vi "使用次数和硬盘序列号.vi"(0 "allowTimes":i32=10, 1 "使用期限":timestamp=timestamp(3494953806 s since 1904-01-01), 2 "serialNum":string, 3 "最小日期":timestamp=timestamp(3494953806 s since 1904-01-01)) -> (7 "curTimes":i32=1000, 8 "writen":bool, 9 "moreTimes":bool, 10 "moreUse":bool)   [LabVIEW 2010]
doc: "This example demonstrates how to write, read, and delete a sample key from the Windows registry. It will not affect the registry in any other way."
uses:
  <vilib>/registry/registry.llb/Registry RtKey.ctl
  <vilib>/registry/registry.llb/Read Registry Value Simple STR.vi
  <vilib>/registry/registry.llb/Write Registry Value Simple STR.vi
  kernel32.dll
  hdd/GetHW.dll
panel:
  out "CPU Manufacturers":string
  out "CPU Specification":string
  out "CPU SN":string
  out "错误输出 3":errorcluster caption="错误输出"
  out "最小日期":bool
  out "未超过使用期限":bool
  out "当前时间":timestamp
  out "Sample Key Deleted?":bool
  in  "清空注册表记录":bool
  out "same":bool
  out "error out":errorcluster caption="错误输出"
  out "硬盘序列号":string
  out "数值 3":i32=12
  out "数值":i32=12
  out "return type":string
  out "已经使用次数":string="My String"
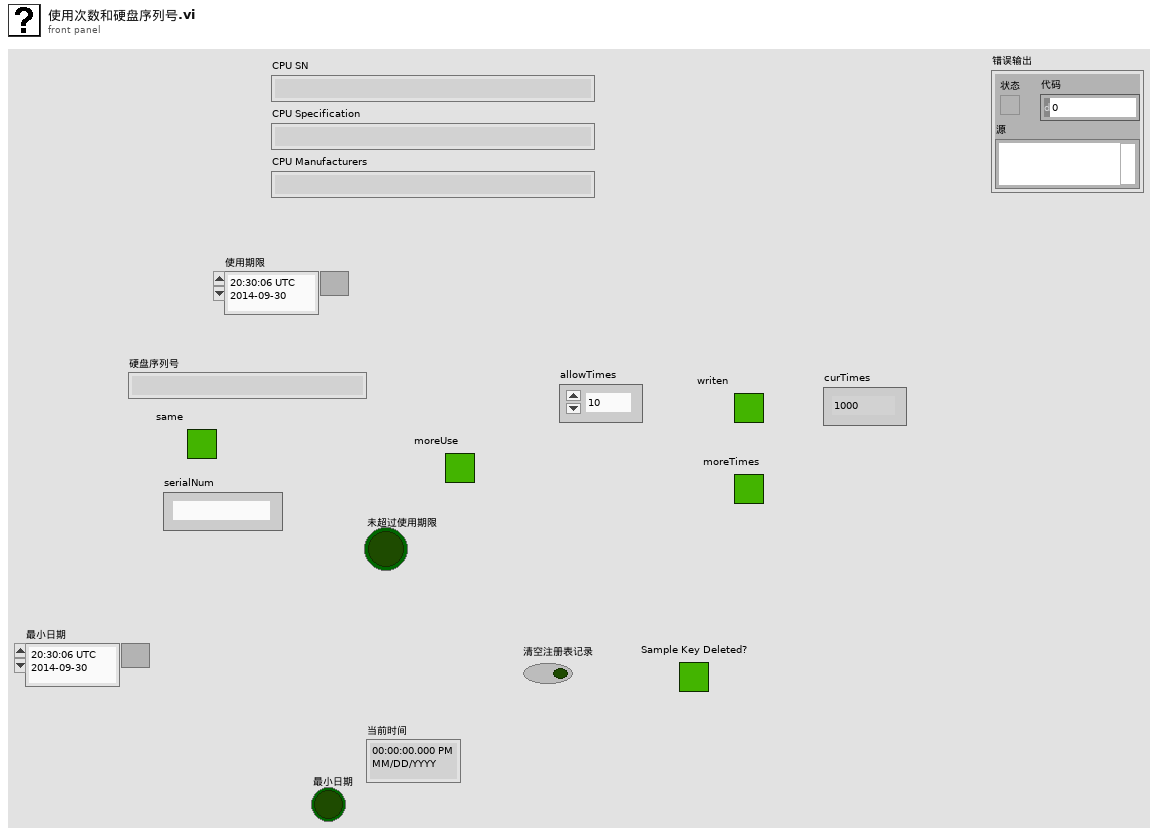
[diagram p1: front panel]
types:
  T1 = typedef "Registry RtKey.ctl" = enum32{"HKEY_CLASSES_ROOT", "HKEY_CURRENT_USER", "HKEY_LOCAL_MACHINE", "HKEY_USERS", "HKEY_PERFORMANCE_DATA", "HKEY_CURRENT_CONFIG", "HKEY_DYN_DATA"}
  T2 = typedef "Registry refnum.ctl" = refnum<k1>
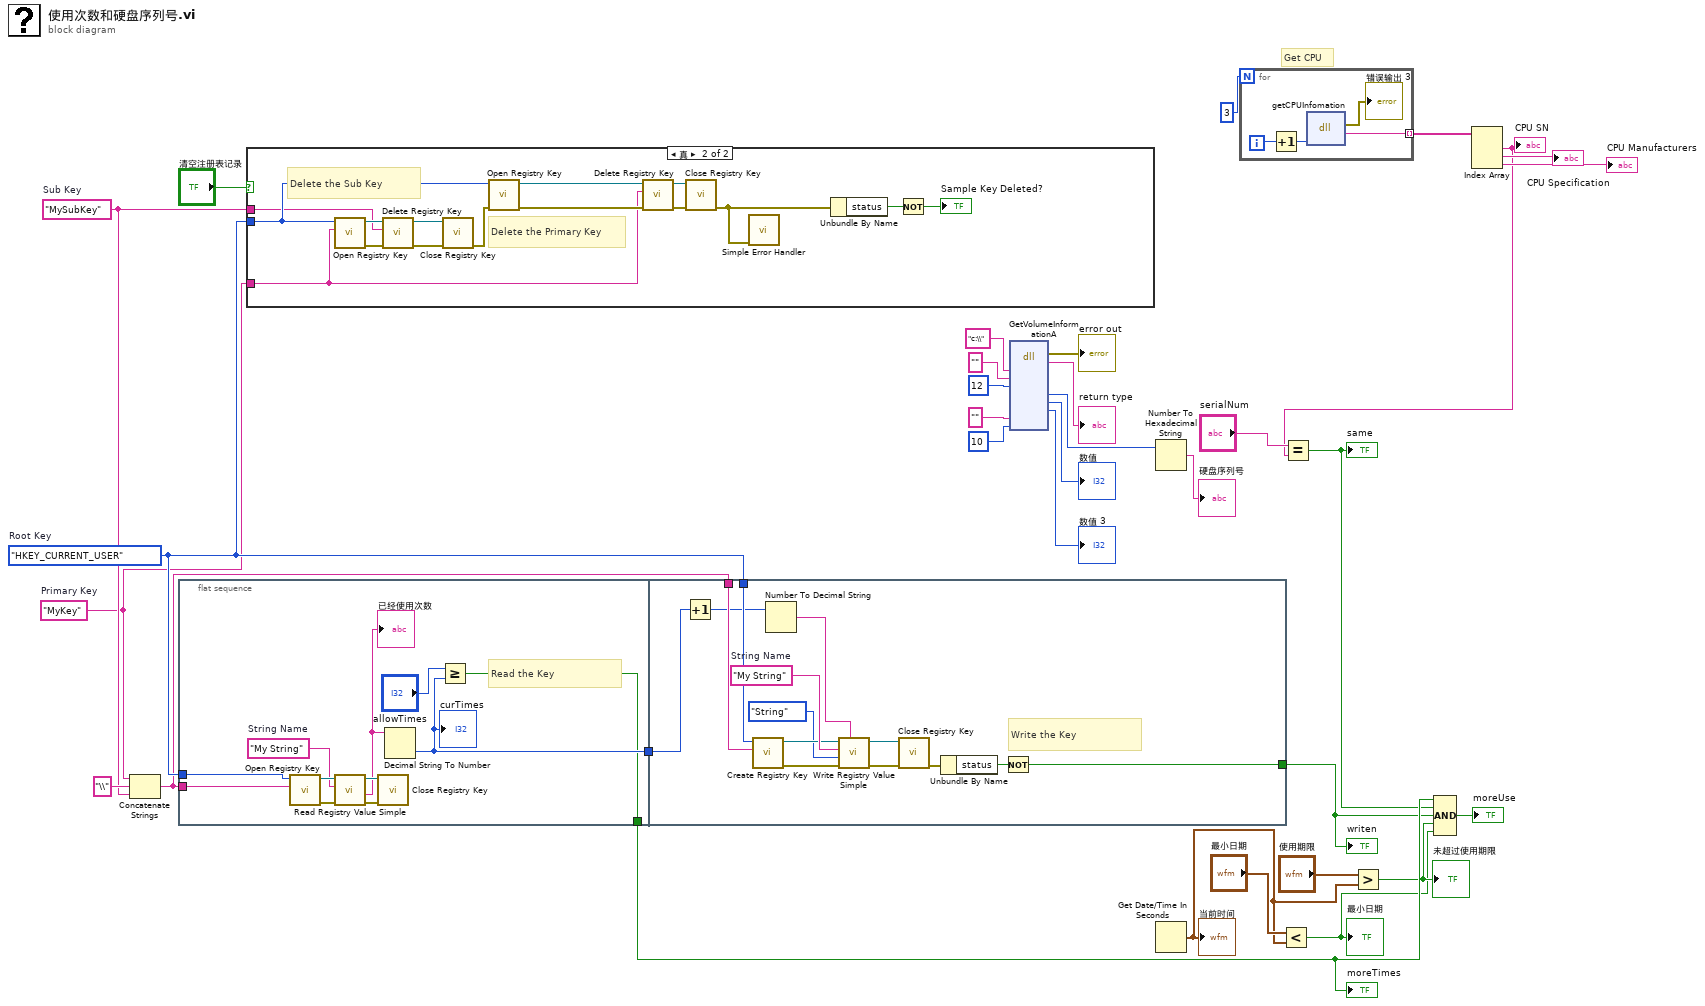
[diagram p0: block diagram]
diagram:
  w15 = "MySubKey"  # Sub Key
  w13 = "MyKey"  # Primary Key
  w17 = Registry_RtKey."HKEY_CURRENT_USER"  # Root Key
  # "Get CPU"
  n1 = Concatenate Strings(w13, "\\", w15) -> (w14:string)
  n2 = flat-sequence {
    tunnel: w17 -> [w39]
    tunnel: w14 -> [w38]
    tunnel: [w35] -> w33
    tunnel: [w34] -> w21
    tunnel: w33 -> [w58]
    tunnel: w14 -> [w50]
    tunnel: w17 -> [w49]
    tunnel: [w46] -> w18
    frame #0 {
      w40 = "My String"  # String Name
      # "Read the Key"
      n3 = call <vilib>:"Open Registry Key.vi"("subkey"=w38, "root key (HKEY_LOCAL_MACHINE)"=w39) -> ("error out"=w41:errorcluster, "refnum out"=w42:T2)  [unwired: 8 in]
      n4 = call-poly <vilib>:"Read Registry Value Simple.vi"("error in (no error)"=w41, "value"=w40, "refnum"=w42) -> ("error out"=w44:errorcluster, "String/Binary data"=w36:string, "refnum out"=w43:T2)  [unwired: 3 in, 1 out]
      "已经使用次数" <- w36
      n5 = call <vilib>:"Close Registry Key.vi"("error in (no error)"=w44, "refnum"=w43) -> ()  [unwired: 5 in, 1 out]
      n6 = Decimal String To Number(string=w36) -> (number=w35:i32)  [unwired: 2 in, 1 out]
      "curTimes" <- w35
      n7 = Greater Or Equal?(x="allowTimes", y=w35) -> (x >= y?=w34:bool)
    }
    frame #1 {
      w57 = "My String"  # String Name
      # "Write the Key"
      n8 = Increment(x=w58) -> (x+1=w48:i32)
      n9 = call <vilib>:"Create Registry Key.vi"("subkey"=w50, "root key (HKEY_LOCAL_MACHINE)"=w49) -> ("error out"=w53:errorcluster, "refnum out"=w55:T2)  [unwired: 7 in, 1 out]
      n10 = Number To Decimal String(number=w48) -> (decimal integer string=w47:string)  [unwired: 1 in]
      n11 = call-poly <vilib>:"Write Registry Value Simple.vi"("String/Binary data"=w47, "error in (no error)"=w53, "simple data type"=enum16{"String", "Binary", "DWORD"}."String", "value"=w57, "refnum"=w55) -> ("error out"=w51:errorcluster, "refnum out"=w52:T2)  [unwired: 3 in]
      n12 = call <vilib>:"Close Registry Key.vi"("error in (no error)"=w51, "refnum"=w52) -> ("error out"=w56:errorcluster)  [unwired: 5 in]
      n13 = Unbundle By Name(w56) -> ("status"=w45:bool)
      n14 = Not(x=w45) -> (.not. x?=w46:bool)
    }
  }
  n15 = case shown="真" "清空注册表记录" {
    tunnel: w17 -> [_ w61]
    tunnel: w13 -> [_ w62]
    tunnel: w15 -> [_ w60]
    frame False {
    }
    frame True {
      # "Delete the Primary Key"
      # "Delete the Sub Key"
      n16 = call <vilib>:"Open Registry Key.vi"("subkey"=w62, "root key (HKEY_LOCAL_MACHINE)"=w61) -> ("error out"=w63:errorcluster, "refnum out"=w64:T2)  [unwired: 8 in]
      n17 = call <vilib>:"Delete Registry Key.vi"("error in (no error)"=w63, "subkey"=w60, "refnum"=w64) -> ("error out"=w65:errorcluster, "refnum out"=w66:T2)  [unwired: 7 in]
      n18 = call <vilib>:"Close Registry Key.vi"("error in (no error)"=w65, "refnum"=w66) -> ("error out"=w71:errorcluster)  [unwired: 5 in]
      n19 = call <vilib>:"Open Registry Key.vi"("error in (no error)"=w71, "root key (HKEY_LOCAL_MACHINE)"=w61) -> ("error out"=w70:errorcluster, "refnum out"=w69:T2)  [unwired: 8 in]
      n20 = call <vilib>:"Delete Registry Key.vi"("error in (no error)"=w70, "subkey"=w62, "refnum"=w69) -> ("error out"=w72:errorcluster, "refnum out"=w73:T2)  [unwired: 7 in]
      n21 = call <vilib>:"Close Registry Key.vi"("error in (no error)"=w72, "refnum"=w73) -> ("error out"=w68:errorcluster)  [unwired: 5 in]
      n22 = call <vilib>:"Simple Error Handler.vi"("error in (no error)"=w68) -> ()  [unwired: 4 in, 5 out]
      n23 = Unbundle By Name(w68) -> ("status"=w59:bool)
      n24 = Not(x=w59) -> (.not. x?=→"Sample Key Deleted?":bool)
    }
  }
  n25 = dll-call lib="kernel32.dll" fn="GetVolumeInformationA"("lpRootPathName"="c:\\", "lpRootPathName"="", "nVolumeNameSize"=12, "lpFileSystemNameBuffer"="", "nFileSystemNameSize"=10) -> (error out=→"error out":errorcluster, "return type"=→"return type":string, "VolumeSerialNumber"=w24:i32, "MaximumComponentLength"=→"数值":i32, "FileSystemFlags"=→"数值 3":i32)  [unwired: 11 in, 1 out]
  n26 = Number To Hexadecimal String(2:w24) -> (0:→"硬盘序列号":string)  [unwired: 1 in]
  n27 = Get Date/Time In Seconds() -> (seconds since 1Jan1904=w7:timestamp)
  "当前时间" <- w7
  n28 = for {
    N: 3 -> [_]
    tunnel: [w75] -> w5 mode=indexing
    i -> [w77]
    n29 = Increment(x=w77) -> (x+1=w76:i32)
    n30 = dll-call lib="C:/Users/cola-pc/Desktop/hdd/GetHW.dll" fn="getCPUInfomation"("infoID"=w76) -> (error out=→"错误输出 3":errorcluster, "return type"=w75:string)  [unwired: 4 in, 1 out]
  }
  n31 = Less?(x="最小日期", y=w7) -> (x < y?=w8:bool)
  "最小日期" <- w8
  n32 = Greater?(x="使用期限", y=w7) -> (0:w10:bool)
  "未超过使用期限" <- w10
  n33 = Index Array(array=w5) -> (element #1=w1:string, element #2=→"CPU Specification":string, element #3=→"CPU Manufacturers":string)  [unwired: 3 in]
  "CPU SN" <- w1
  n34 = Equal?(x="serialNum", y=w1) -> (x = y?=w20:bool)
  "same" <- w20
  n35 = Compound Arithmetic op=AND(w21, w20, w18, w10, w8) -> (→"moreUse":bool)
  "moreTimes" <- w21
  "writen" <- w18
